vi "InsertNewRequest.vi"(8 "error in":errorcluster, 10 "RequestID":u32) -> (0 "error out":errorcluster)   [LabVIEW 2015]
uses:
  TypeDef/RequestsTableDbTableName.ctl
  TypeDef/RequestsTableColumnNames.ctl
  TypeDef/RequestTableCluster.ctl
  <vilib>/addons/database/Connection.llb/DB Tools Open Connec (Path).vi
  <vilib>/addons/database/NI_Database_API.lvlib
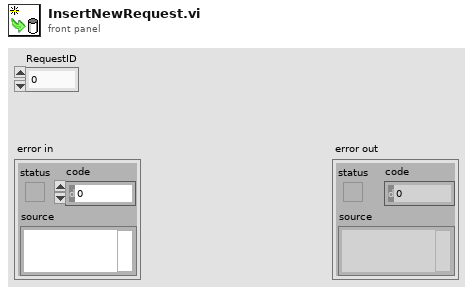
[diagram p1: front panel]
types:
  T1 = typedef "RequestTableCluster.ctl" = cluster{"RequestID":u32, "PersonnelType":enum16{"Dr", "Nurse"}, "StartTime":timestamp, "StartName":string, "AckTime":timestamp, "AckName":string, "FulfilledTime":timestamp, "FulfilledName":string}
  T2 = typedef "RequestsTableColumnNames.ctl" = string[]
  T3 = typedef "RequestsTableDbTableName.ctl" = string
  T4 = typedef "NI_Database_API.lvlib/Conn ObjectReference.ctl" = refnum<k1>
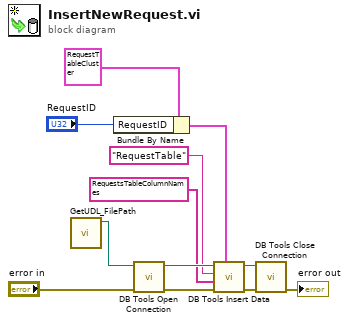
[diagram p0: block diagram]
diagram:
  n1 = call "GetUDL_FilePath.vi"() -> ("UDL file path"=w12:path)  [unwired: 11 in]
  n2 = Bundle By Name(cluster=T1 {"RequestID"=0, "PersonnelType"=enum."Dr", "StartTime"=timestamp(0 s since 1904-01-01), "StartName"="", "AckTime"=timestamp(0 s since 1904-01-01), "AckName"="", "FulfilledTime"=timestamp(0 s since 1904-01-01), "FulfilledName"=""} ("RequestTable"), "RequestID"="RequestID") -> (w4:T1)
  n3 = call-poly <vilib>:"DB Tools Open Connection.vi"("error in (no error)"="error in", "connection information"=w12) -> ("error out"=w8:errorcluster, "connection reference"=w9:T4)  [unwired: 6 in]
  n4 = call <vilib>:"DB Tools Insert Data.vi"("data"=w4, "error in (no error)"=w8, "columns"=T2 ["RequestID", "PersonnelType", "StartTime", "StartName", "AckTime", "AckName", "FulfilledTime", "FulfilledName"] ("Array"), "table"=T3 "RequestTable", "connection reference"=w9) -> ("error out"=w10:errorcluster, "connection reference out"=w11:T4)  [unwired: 5 in]
  n5 = call <vilib>:"DB Tools Close Connection.vi"("error in (no error)"=w10, "connection reference"=w11) -> ("error out"=→"error out":errorcluster)  [unwired: 5 in]
